vi "solar_write ThisData.vi"(8 "error in (no error)":errorcluster, 10 "Data":variant, 11 "solar in":refnum<class "solar.lvclass">) -> (0 "error out":errorcluster, 3 "solar out":refnum<class "solar.lvclass">)   [LabVIEW 2018, in "solar.lvclass"]
doc: "This sets the targets shared variant data. The shared data is stored in a Data Value Reference for each target. Use this target data to share data globally throughout the SOLAR application."
uses:
  solar.lvclass
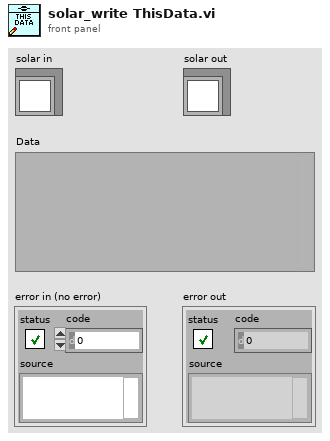
[diagram p1: front panel]
types:
  T1 = typedef "solar_ctl SOLAR Refnum.ctl" = refnum<k1>
  T2 = typedef "solar_ctl SOLAR Global.ctl" = cluster{"Targets":T3[], "AppDir":path, "solar.ini":path, "ConfigsDir":path, "CosmosDir":path, "LogsDir":path, "ExePath":path, "ExeVersion":string, "PartNum":string, "AppSetup":string, "Title":string, "Main.ini":path, "Temp.ini":path, "vSOLAR":string, "Splash.png":string, "SplashWait":i32, "SOLARUE":refnum<user-event>, "VoyagerRefnum":T4, "QTimerRefnum":T5}
  T3 = typedef "solar_ctl Target Global.ctl" = cluster{"Target":string, "Q":refnum<queue>, "UE":refnum<user-event>, "VI":refnum<vi>, "Menu":refnum<k9>, "Data":refnum<data-value>, "Attributes":variant}
  T4 = typedef "solar_voy_ctl Voyager Refnum.ctl" = refnum<k1>
  T5 = typedef "solar_qtimer_ctl Refnum.ctl" = refnum<k1>
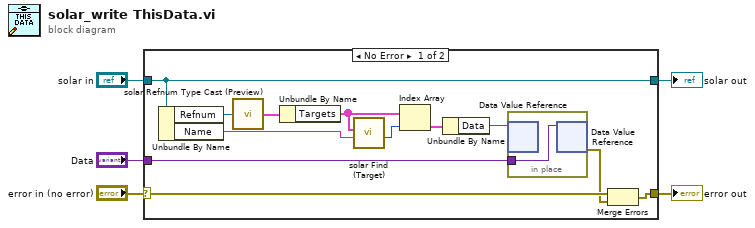
[diagram p0: block diagram]
diagram:
  n1 = case shown="No Error" "error in (no error)" {
    selector: "error in (no error)" -> [w17 w20]
    tunnel: "solar in" -> [w10 w19]
    tunnel: [w7 w20] -> w3
    tunnel: [w10 w19] -> w4
    tunnel: "Data" -> [w8 _]
    frame No Error {
      n2 = Unbundle By Name(w10) -> ("Refnum"=w13:T1, "Name"=w16:string)
      n3 = call "solar Refnum Type Cast (Preview).vi"("Refnum"=w13) -> ("SOLAR"=w12:T2)  [unwired: 8 in]
      n4 = Unbundle By Name(w12) -> ("Targets"=w14:T3[])
      n5 = call "solar Find (Target).vi"("Target"=w16, "Targets"=w14) -> ("Target Index"=w15:i32)  [unwired: 8 in, 1 out]
      n6 = Index Array(array=w14, index=w15) -> (element=w11:T3)
      n7 = Unbundle By Name(w11) -> ("Data"=w9:refnum<data-value>)
      n8 = in-place {
        in-place-border: w8 -> [w18]
        n9 = in-place-dvr #1(w9) -> ()  [unwired: 2 out]
        n10 = in-place-dvr #1(w18) -> (w6:errorcluster)  [unwired: 1 out]
      }
      n11 = Merge Errors(w17, w6) -> (w7:errorcluster)
    }
    frame Error {
    }
  }
  "error out" <- w3
  "solar out" <- w4
